vi "Push.vi"(6 "Debug":T1 {"Time" format="%<%H:%M:%S%3u>T"}, 8 "error in (no error)":errorcluster, 9 "ID":i32) -> (0 "error out":errorcluster)   [LabVIEW 2022 SP3, in "Error.lvlib"]
uses:
  Error.lvlib
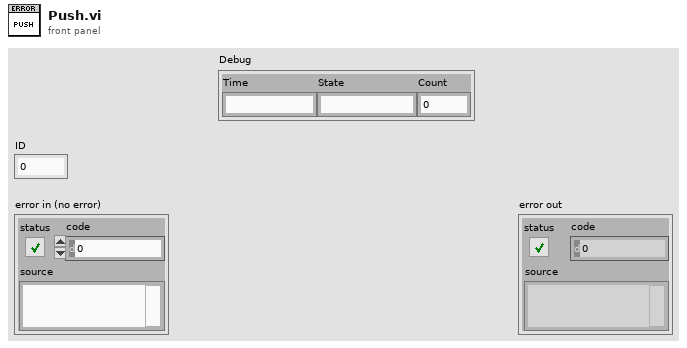
[diagram p1: front panel]
types:
  T1 = cluster{"Time":timestamp, "State":string, "Count":u32}
  T2 = cluster{"Error":errorcluster, "ID":i32, "Debug":cluster{"Time":timestamp, "State":string, "Count":u32}}
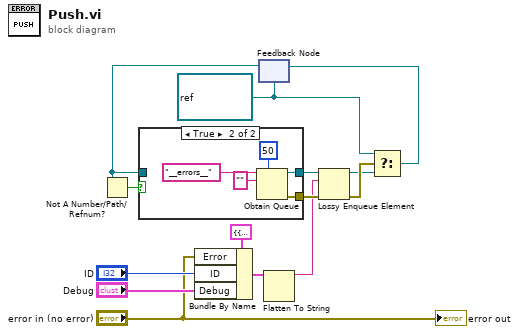
[diagram p0: block diagram]
diagram:
  w1 = refnum<queue> refnum ("queue out")
  n1 = Bundle By Name(cluster=T2 {"Error"={"status"=FALSE, "code"=0, "source"=""}, "ID"=0, "Debug"={"Time"=timestamp(0 s since 1904-01-01), "State"="", "Count"=0}} ("Error"), "Error"="error in (no error)", "ID"="ID", "Debug"="Debug") -> (w6:T2)
  n2 = feedback #1(w1) -> (w14:refnum<queue>)
  n3 = Not A Number/Path/Refnum?(number/path/refnum=w14) -> (NaN/Path/Refnum?=w13:bool)
  n4 = case shown="True" w13 {
    tunnel: [w15 w19] -> w12
    tunnel: w14 -> [w15 _]
    tunnel: [_ w16] -> w8
    frame False {
    }
    frame True {
      n5 = Obtain Queue(max queue size (-1, unlimited)=50, name (unnamed)="__errors__", element data type="") -> (queue out=w19:refnum<queue>, error out=w16:errorcluster)  [unwired: 2 in, 1 out]
    }
  }
  n6 = Flatten To String(anything=w6) -> (data string=w5:string)  [unwired: 3 in, 2 out]
  n7 = Lossy Enqueue Element(queue=w12, element=w5, error in (no error)=w8) -> (queue out=w3:refnum<queue>, error out=w4:errorcluster)  [unwired: 2 out]
  n8 = Select(t=w1, s=w4, f=w3) -> (s? t:f=w2:refnum<queue>)
  n9 = feedback-in #1(w2) -> ()
  "error out" <- "error in (no error)"
